vi "Example -- Producer-Consumer as a Stack (FILO).vi"() -> ()   [LabVIEW 2013]
uses:
  VariantBuffer/buffer-type -- enum.ctl
  VariantBuffer/VariantBuffer.lvclass
panel:
  out "Processing...":string
  in  "Trigger":bool
  out "Stack":string[](array[string])
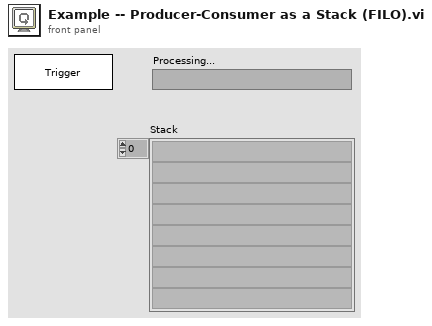
[diagram p1: front panel]
types:
  T1 = typedef "CircularBuffer.lvlib/VariantBuffer.lvclass/buffer-type -- enum.ctl" = enum16{"Queue", "Stack"}
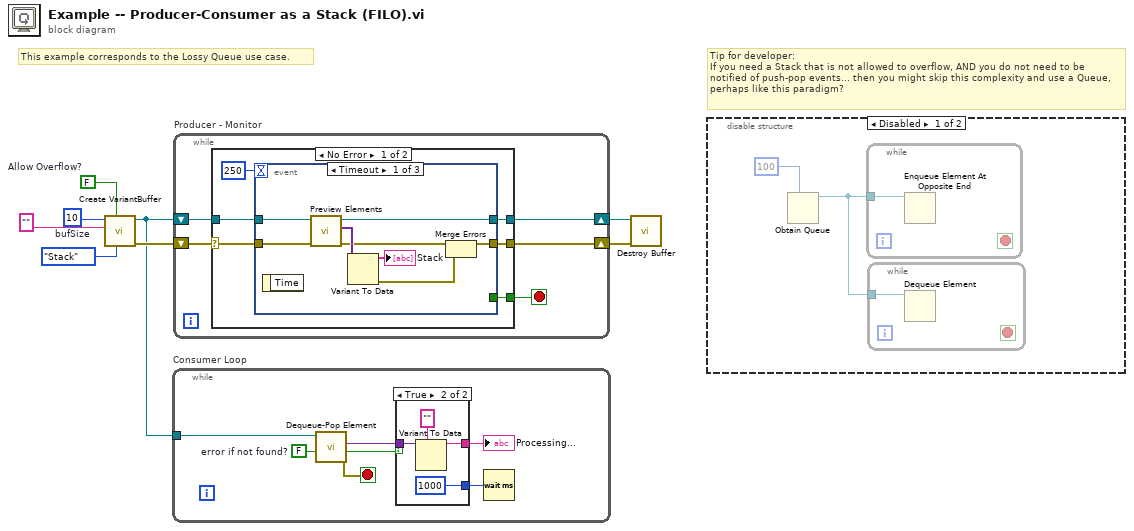
[diagram p0: block diagram]
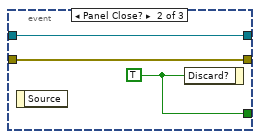
[diagram p3: hidden frame]
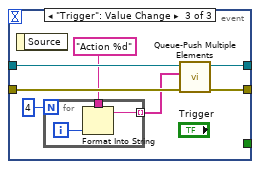
[diagram p4: hidden frame]
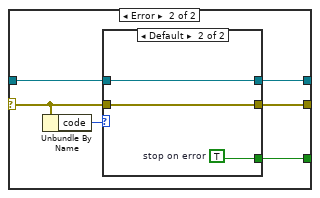
[diagram p5: hidden frame]
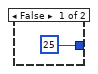
[diagram p7: hidden frame]
diagram:
  w1 = FALSE  # Allow Overflow?
  w8 = 10  # bufSize
  # "Tip for developer: \nIf you need a Stack that is not allowed to overflow, AND you do not need to be notified of push-pop events... then you might skip this complexity and use a Queue, perhaps like this paradigm?"
  # "This example corresponds to the Lossy Queue use case."
  n1 = call "Create VariantBuffer.vi"("buffer-type"=buffer-type_--_enum."Stack", "Allow Overflow?"=w1, "default"="", "bufSize"=w8) -> ("error out"=w5:errorcluster, "Buffer"=w3:refnum<data-value>)  [unwired: 6 in]
  n2 = while "Consumer Loop" {
    tunnel: w3 -> [w15]
    stop <- w9 stop-if-true
    w12 = FALSE  # error if not found?
    n3 = call "Dequeue-Pop Element.vi"("error if not found?"=w12, "Buffer in"=w15) -> ("error out"=w9:errorcluster, "found"=w11:bool, "element"=w14:variant)  [unwired: 5 in, 2 out]
    n4 = case shown="True" w11 {
      tunnel: w14 -> [_ w20]
      tunnel: [_ w19] -> w13
      tunnel: [u32 25 ("milliseconds to wait") u32 1000 ("milliseconds to wait")] -> w10
      frame False {
      }
      frame True {
        n5 = Variant To Data(type="", Variant=w20) -> (data=w19:string)  [unwired: 1 in, 1 out]
      }
    }
    "Processing..." <- w13
    n6 = Wait (ms)(milliseconds to wait=w10) -> ()  [unwired: 1 out]
  }
  n7 = while "Producer - Monitor" {
    shift-right: [w24] -> w6
    shift-left: w3 -> [w25]
    shift-right: [w23] -> w4
    shift-left: w5 -> [w21]
    stop <- w22 stop-if-true
    n8 = case shown="No Error" w21 {
      selector: w21 -> [w26 w54]
      tunnel: w25 -> [w30 w55]
      tunnel: [w29 w56] -> w24
      tunnel: [w28 w53] -> w23
      tunnel: [w27 w58] -> w22
      frame No Error {
        n9 = event shown="[0] Timeout" {
          selector: _ -> [_ _ _]
          dyn-events: _ -> [_ _ _]
          timeout: 250 -> [_ _ _]
          tunnel: w30 -> [w39 w42 w49]
          tunnel: [w38 w42 w48] -> w29
          tunnel: [_ w41 _] -> w27
          tunnel: w26 -> [w35 w40 w47]
          tunnel: [w34 w40 w46] -> w28
          event Timeout {
            n10 = event-data() -> ()  [unwired: 1 in, 1 out]
            n11 = call "Preview Elements.vi"("error in"=w35, "ByteBuffer in"=w39) -> ("error out"=w33:errorcluster, "elements"=w36:variant[], "ByteBuffer"=w38:refnum<data-value>)  [unwired: 7 in]
            n12 = Variant To Data(Variant=w36) -> (data=→"Stack":string[], error out=w32:errorcluster)  [unwired: 2 in]
            n13 = Merge Errors(w33, w32) -> (w34:errorcluster)
          }
          event Panel Close? {
            w41 = TRUE ("Discard?")
            n14 = event-data() -> ()  [unwired: 1 in, 1 out]
            n15 = event-data("Discard?"=w41) -> ()  [unwired: 1 in, 1 out]
          }
          event "Trigger": Value Change {
            n16 = event-data() -> ()  [unwired: 1 in, 1 out]
            n17 = for {
              N: 4 -> [_]
              tunnel: "Action %d" -> [w51]
              tunnel: [w50] -> w43 mode=indexing
              i -> [w52]
              n18 = Format Into String(format string=w51, w52) -> (resulting string=w50:string)  [unwired: 2 in, 1 out]
            }
            n19 = call "Queue-Push Multiple Elements.vi"("error in"=w47, "elements"=w43, "Buffer in"=w49) -> ("error out"=w46:errorcluster, "Buffer"=w48:refnum<data-value>)  [unwired: 6 in, 1 out]
          }
        }
      }
      frame Error {
        n20 = Unbundle By Name(w54) -> ("code"=w57:i32)
        n21 = case shown="Default" w57 {
          tunnel: [_ w62] -> w58
          tunnel: [w59 w61] -> w56
          tunnel: w55 -> [w59 w61]
          tunnel: w54 -> [_ w60]
          tunnel: [_ w60] -> w53
          frame 0 {
            # "Handle Error\n& Continue"
          }
          frame Default {
            w62 = TRUE  # stop on error
          }
        }
      }
    }
  }
  n22 = call "Destroy Buffer.vi"("error in"=w4, "Buffer"=w6) -> ()  [unwired: 8 in, 2 out]
  n23 = disable-structure shown="Disabled" {
    frame Disabled {
      n24 = Obtain Queue(max queue size (-1, unlimited)=100) -> (queue out=w63:refnum<queue>)  [unwired: 4 in, 2 out]
      n25 = while {
        tunnel: w63 -> [w66]
        stop <- _ stop-if-true
        n26 = Enqueue Element At Opposite End(queue=w66) -> ()  [unwired: 3 in, 3 out]
      }
      n27 = while {
        tunnel: w63 -> [w65]
        stop <- _ stop-if-true
        n28 = Dequeue Element(queue=w65) -> ()  [unwired: 2 in, 4 out]
      }
    }
    frame Enabled {
    }
  }
